vi "S2C_CMD_FormatParameters.vi"(8 "Error In":errorcluster, 9 "CmdName":string, 10 "Type":string, 11 "Cmd":string) -> (0 "Error Out":errorcluster, 1 "RecReturn?":bool, 2 "Returns":string[](array[string]), 3 "Parameters":string[](array[string]))   [LabVIEW 2015]
doc: "Formats a command input parameter according to its type."
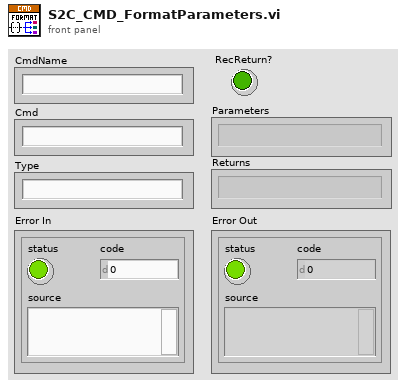
[diagram p1: front panel]
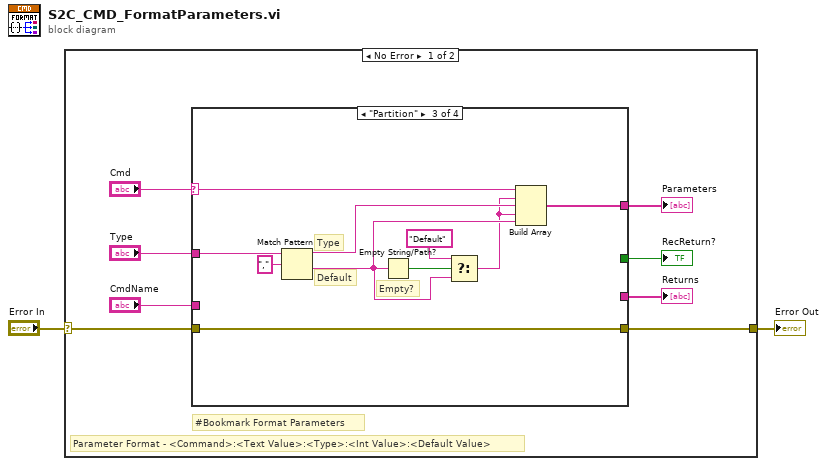
[diagram p0: block diagram]
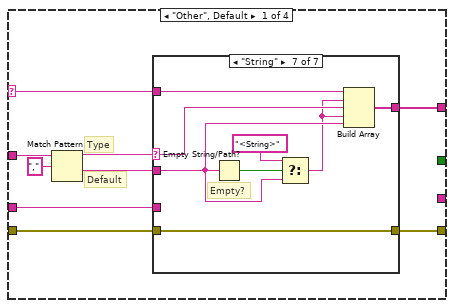
[diagram p2: hidden frame]
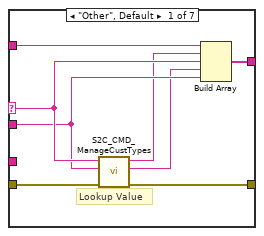
[diagram p3: hidden frame]
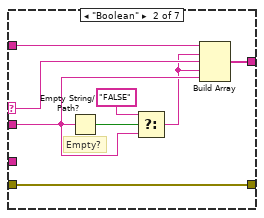
[diagram p4: hidden frame]
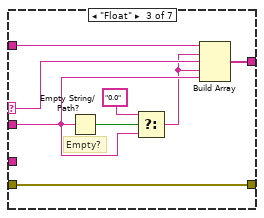
[diagram p5: hidden frame]
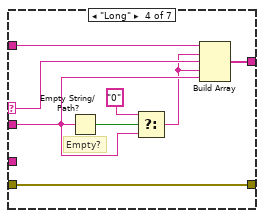
[diagram p6: hidden frame]
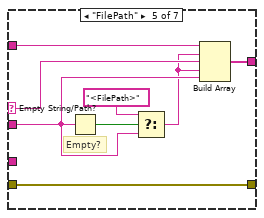
[diagram p7: hidden frame]
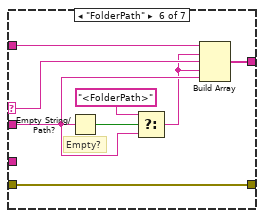
[diagram p8: hidden frame]
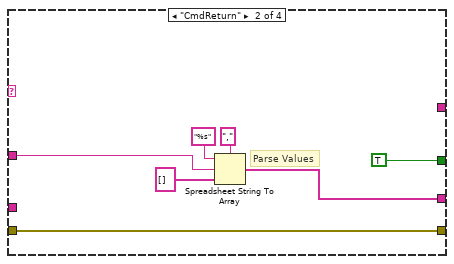
[diagram p9: hidden frame]
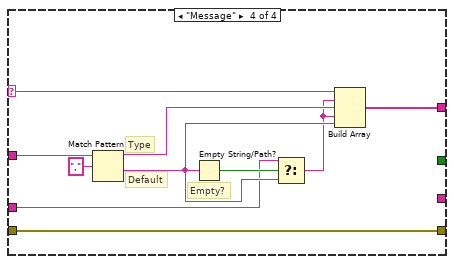
[diagram p10: hidden frame]
diagram:
  n1 = case shown="No Error" "Error In" {
    selector: "Error In" -> [w10 w103]
    tunnel: [w5 w103] -> w1
    frame No Error {
      # "#Bookmark Format Parameters"
      # "Parameter Format - <Command>:<Text Value>:<Type>:<Int Value>:<Default Value>"
      n2 = case shown="\"Partition\"" "Cmd" {
        selector: "Cmd" -> [w18 _ w92 w102]
        tunnel: w10 -> [w19 w82 w90 w100]
        tunnel: "Type" -> [w15 w81 w88 w98]
        tunnel: "CmdName" -> [w11 _ _ w94]
        tunnel: [w17 _ w91 w101] -> w3
        tunnel: [w16 w82 w90 w100] -> w5
        tunnel: [_ w76 _ _] -> w6
        tunnel: [_ TRUE _ _] -> w4
        frame "Other", Default {
          # "Default"
          # "Type"
          n3 = Match Pattern(string=w15, regular expression=",") -> (before substring=w13:string, after substring=w12:string)  [unwired: 1 in, 2 out]
          n4 = case shown="\"String\"" w13 {
            selector: w13 -> [w25 w30 w38 w46 w54 w62 w70]
            tunnel: w19 -> [w24 w35 w43 w51 w59 w67 w75]
            tunnel: w18 -> [w27 w34 w42 w50 w58 w66 w74]
            tunnel: [w26 w33 w41 w49 w57 w65 w73] -> w17
            tunnel: [w23 w35 w43 w51 w59 w67 w75] -> w16
            tunnel: w12 -> [w22 w29 w37 w45 w53 w61 w69]
            tunnel: w11 -> [_ _ _ _ _ _ _]
            frame "Other", Default {
              # "Lookup Value"
              n5 = call "S2C_CMD_ManageCustTypes.vi"("Error In"=w24, "Default"=w22, "Type"=w25) -> ("Error Out"=w23:errorcluster, "Value_Int"=w20:string, "Value_String"=w21:string)  [unwired: 6 in]
              n6 = Build Array(w27, w21, w25, w20, w22) -> (w26:string[])
            }
            frame "Boolean" {
              # "Empty?"
              n7 = Empty String/Path?(string/path=w29) -> (empty?=w32:bool)
              n8 = Select(t="FALSE", s=w32, f=w29) -> (s? t:f=w28:string)
              n9 = Build Array(w34, w28, w30, w28, w29) -> (w33:string[])
            }
            frame "Float" {
              # "Empty?"
              n10 = Empty String/Path?(string/path=w37) -> (empty?=w40:bool)
              n11 = Select(t="0.0", s=w40, f=w37) -> (s? t:f=w36:string)
              n12 = Build Array(w42, w36, w38, w36, w37) -> (w41:string[])
            }
            frame "Long" {
              # "Empty?"
              n13 = Empty String/Path?(string/path=w45) -> (empty?=w48:bool)
              n14 = Select(t="0", s=w48, f=w45) -> (s? t:f=w44:string)
              n15 = Build Array(w50, w44, w46, w44, w45) -> (w49:string[])
            }
            frame "FilePath" {
              # "Empty?"
              n16 = Empty String/Path?(string/path=w53) -> (empty?=w56:bool)
              n17 = Select(t="<FilePath>", s=w56, f=w53) -> (s? t:f=w52:string)
              n18 = Build Array(w58, w52, w54, w52, w53) -> (w57:string[])
            }
            frame "FolderPath" {
              # "Empty?"
              n19 = Empty String/Path?(string/path=w61) -> (empty?=w64:bool)
              n20 = Select(t="<FolderPath>", s=w64, f=w61) -> (s? t:f=w60:string)
              n21 = Build Array(w66, w60, w62, w60, w61) -> (w65:string[])
            }
            frame "String" {
              # "Empty?"
              n22 = Empty String/Path?(string/path=w69) -> (empty?=w72:bool)
              n23 = Select(t="<String>", s=w72, f=w69) -> (s? t:f=w68:string)
              n24 = Build Array(w74, w68, w70, w68, w69) -> (w73:string[])
            }
          }
        }
        frame "CmdReturn" {
          # "Parse Values"
          n25 = Spreadsheet String To Array(delimiter (Tab)=",", format string="%s", spreadsheet string=w81, array type (2D Dbl)=string[] []) -> (array=w76:string[])
        }
        frame "Partition" {
          # "Empty?"
          # "Default"
          # "Type"
          n26 = Match Pattern(string=w88, regular expression=",") -> (before substring=w87:string, after substring=w85:string)  [unwired: 1 in, 2 out]
          n27 = Empty String/Path?(string/path=w85) -> (empty?=w86:bool)
          n28 = Select(t="Default", s=w86, f=w85) -> (s? t:f=w84:string)
          n29 = Build Array(w92, w84, w87, w84, w85) -> (w91:string[])
        }
        frame "Message" {
          # "Empty?"
          # "Default"
          # "Type"
          n30 = Match Pattern(string=w98, regular expression=",") -> (before substring=w97:string, after substring=w95:string)  [unwired: 1 in, 2 out]
          n31 = Empty String/Path?(string/path=w95) -> (empty?=w96:bool)
          n32 = Select(t=w94, s=w96, f=w95) -> (s? t:f=w93:string)
          n33 = Build Array(w102, w93, w97, w93, w95) -> (w101:string[])
        }
      }
      "Parameters" <- w3
      "Returns" <- w6
      "RecReturn?" <- w4
    }
    frame Error {
    }
  }
  "Error Out" <- w1
